vi "Get the closest value.vi"(10 "Voltage":dbl format="%.2g", 11 "Data":dbl[](array[numeric])) -> (3 "Dataout":i32)   [LabVIEW 2010]
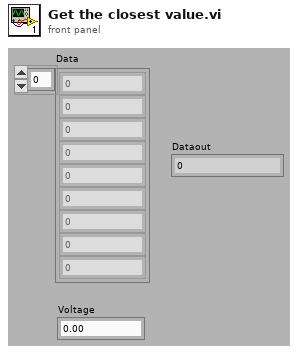
[diagram p1: front panel]
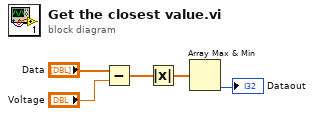
[diagram p0: block diagram]
diagram:
  n1 = Subtract(x="Data", y="Voltage") -> (x-y=w1:dbl[])
  n2 = Absolute Value(x=w1) -> (abs(x)=w2:dbl[])
  n3 = Array Max & Min(array=w2) -> (min index (indices)=→"Dataout":i32)  [unwired: 3 out]
